vi "for_condicional.vi"() -> ()   [LabVIEW 2020]
panel:
  out "Array 2":i32[](array[numeric])
  out "Array":i32[](array[numeric])
  out "Thermometer":dbl(slide) scale=0.0..100.0
  out "Numeric":i32
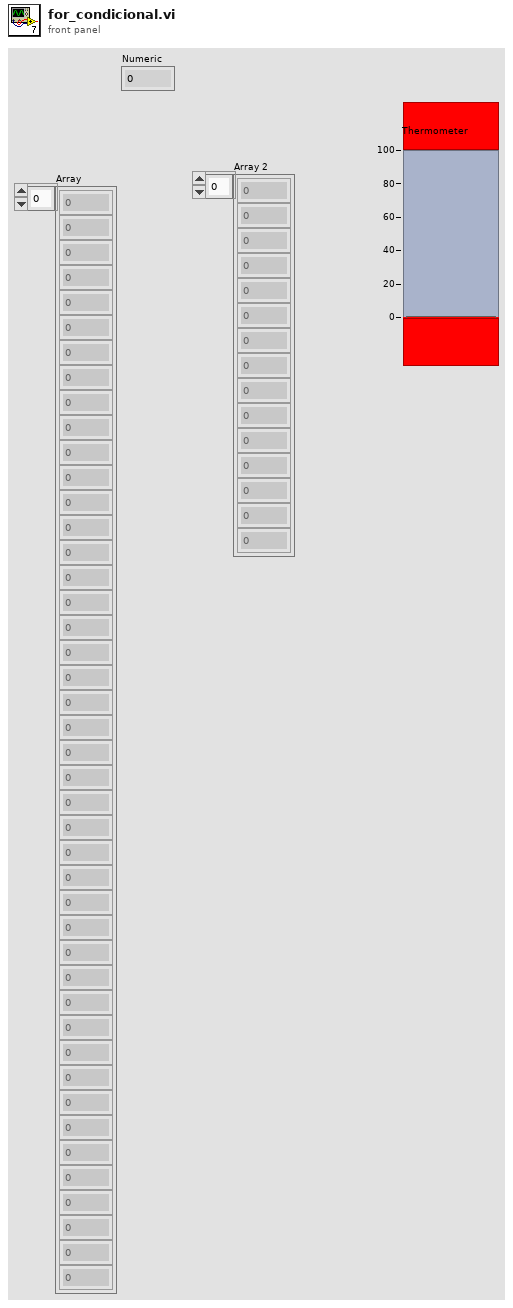
[diagram p1: front panel]
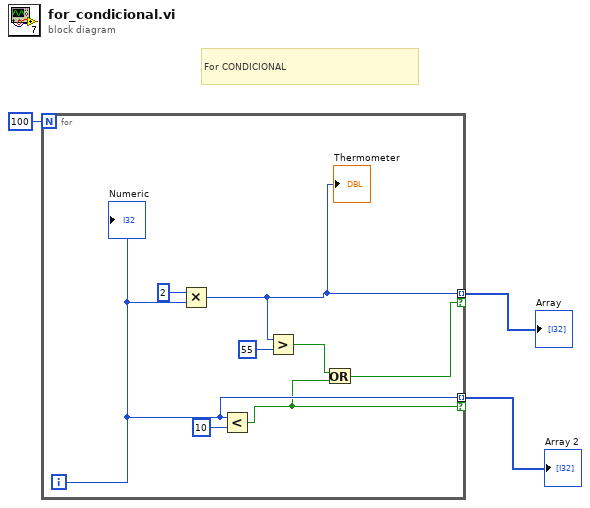
[diagram p0: block diagram]
diagram:
  # "For CONDICIONAL"
  n1 = for {
    N: 100 -> [_]
    tunnel: [w10] -> w2 mode=indexing if=w4
    tunnel: [w7] -> w1 mode=indexing if=w5
    i -> [w7]
    n2 = Multiply(x=2, y=w7) -> (x*y=w10:i32)
    "Thermometer" <- w10
    n3 = Less?(x=w7, y=10) -> (x < y?=w5:bool)
    n4 = Greater?(x=w10, y=55) -> (0:w6:bool)
    n5 = Or(x=w6, y=w5) -> (x .or. y?=w4:bool)
    "Numeric" <- w7
  }
  "Array" <- w2
  "Array 2" <- w1
